vi "SolveMotor_Volts,Current.vi"(8 "Reference Voltage (12)":dbl=12.0, 9 "Motor Characteristics":T2, 10 "Motor Current":dbl, 11 "Motor Voltage":dbl) -> (3 "Motor Data":T1)   [LabVIEW 2014]
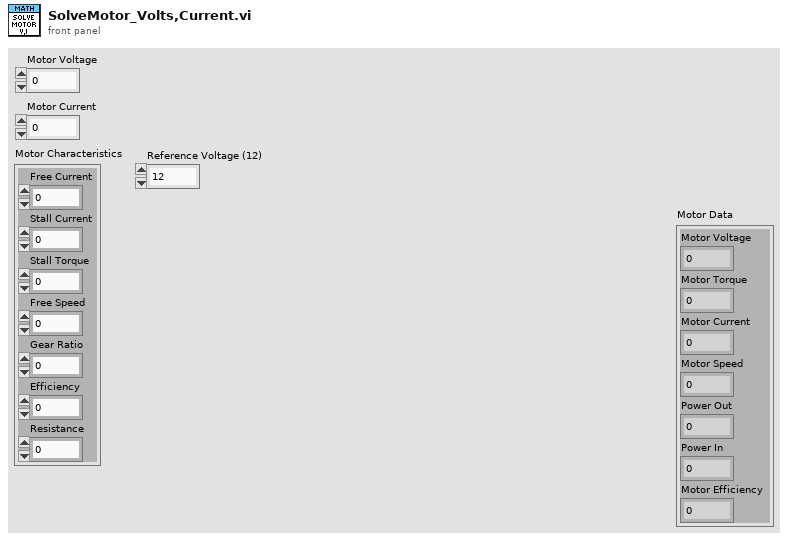
[diagram p1: front panel]
types:
  T1 = cluster{"Motor Voltage":dbl, "Motor Torque":dbl, "Motor Current":dbl, "Motor Speed":dbl, "Power Out":dbl, "Power In":dbl, "Motor Efficiency":dbl}
  T2 = cluster{"Free Current":dbl, "Stall Current":dbl, "Stall Torque":dbl, "Free Speed":dbl, "Gear Ratio":dbl, "Efficiency":dbl, "Resistance":dbl}
  T3 = cluster{"[0]":dbl, "[1]":dbl, "[2]":dbl, "[3]":dbl, "[4]":dbl, "[5]":dbl, "[6]":dbl}
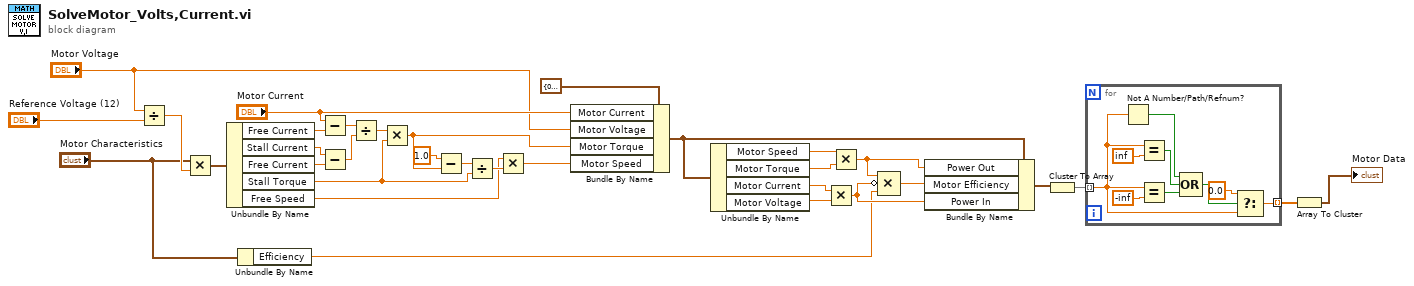
[diagram p0: block diagram]
diagram:
  n1 = Divide(x="Motor Voltage", y="Reference Voltage (12)") -> (x/y=w32:dbl)
  n2 = Multiply(x="Motor Characteristics", y=w32) -> (x*y=w23:T2)
  n3 = Unbundle By Name(w23) -> ("Free Current"=w31:dbl, "Stall Current"=w29:dbl, "Free Current"=w30:dbl, "Stall Torque"=w19:dbl, "Free Speed"=w17:dbl)
  n4 = Unbundle By Name("Motor Characteristics") -> ("Efficiency"=w5:dbl)
  n5 = Subtract(x="Motor Current", y=w31) -> (x-y=w28:dbl)
  n6 = Subtract(x=w29, y=w30) -> (x-y=w27:dbl)
  n7 = Divide(x=w28, y=w27) -> (x/y=w26:dbl)
  n8 = Multiply(x=w26, y=w19) -> (x*y=w21:dbl)
  n9 = Subtract(x=1.0, y=w21) -> (x-y=w20:dbl)
  n10 = Divide(x=w20, y=w19) -> (x/y=w18:dbl)
  n11 = Multiply(x=w17, y=w18) -> (x*y=w16:dbl)
  n12 = Bundle By Name(cluster=T1 {"Motor Voltage"=0.0, "Motor Torque"=0.0, "Motor Current"=0.0, "Motor Speed"=0.0, "Power Out"=0.0, "Power In"=0.0, "Motor Efficiency"=0.0} ("Motor Data 2"), "Motor Current"="Motor Current", "Motor Voltage"="Motor Voltage", "Motor Torque"=w21, "Motor Speed"=w16) -> (w7:T1)
  n13 = Unbundle By Name(w7) -> ("Motor Speed"=w15:dbl, "Motor Torque"=w14:dbl, "Motor Current"=w12:dbl, "Motor Voltage"=w13:dbl)
  n14 = Multiply(x=w12, y=w13) -> (x*y=w9:dbl)
  n15 = Multiply(x=w15, y=w14) -> (x*y=w10:dbl)
  n16 = Compound Arithmetic op=MULTIPLY(w10, invert w9, w5) -> (w11:dbl)
  n17 = Bundle By Name(cluster=w7, "Power Out"=w10, "Motor Efficiency"=w11, "Power In"=w9) -> (w2:T1)
  n18 = Cluster To Array(cluster=w2) -> (array=w4:dbl[])
  n19 = for {
    tunnel: w4 -> [w39] mode=indexing
    tunnel: [w34] -> w3 mode=indexing
    n20 = Not A Number/Path/Refnum?(number/path/refnum=w39) -> (NaN/Path/Refnum?=w38:bool)
    n21 = Equal?(x=w39, y=inf) -> (x = y?=w36:bool)
    n22 = Equal?(x=w39, y=-inf) -> (x = y?=w37:bool)
    n23 = Compound Arithmetic op=OR(w38, w36, w37) -> (w35:bool)
    n24 = Select(t=0.0, s=w35, f=w39) -> (s? t:f=w34:dbl)
  }
  n25 = Array To Cluster(array=w3) -> (cluster=→"Motor Data":T3)
